vi "BitShifting.vi"(11 "register in":u16) -> (0 "4-1 Error":bool, 1 "8-5 Error":bool, 2 "12-9 Error":bool, 3 "16-13 Error":bool, 4 "SystemFault":bool, 5 "Warning":bool)   [LabVIEW 2014]
panel:
  out "16-13":u8
  out "12-9":u8
  out "8-5":u8
  out "1-4":u8
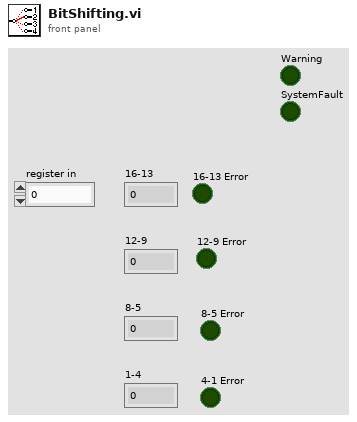
[diagram p1: front panel]
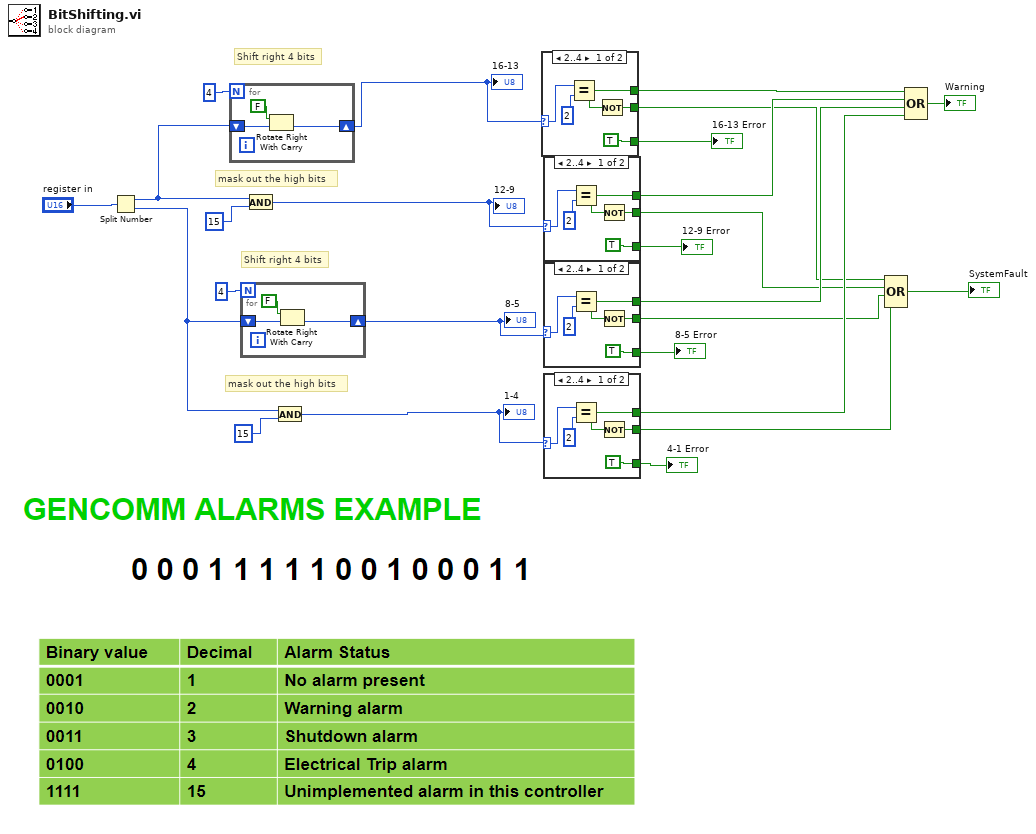
[diagram p0: block diagram]
diagram:
  # "mask out the high bits"
  # "Shift right 4 bits"
  # "mask out the high bits"
  # "Shift right 4 bits"
  n1 = Split Number(x="register in") -> (hi(x)=w21:u8, lo(x)=w25:u8)
  n2 = for {
    N: 4 -> [_]
    shift-right: [w27] -> w17
    shift-left: w21 -> [w28]
    n3 = Rotate Right With Carry(2:w28, 3:FALSE ("carry")) -> (0:w27:u8)  [unwired: 1 out]
  }
  "16-13" <- w17
  n4 = for {
    N: 4 -> [_]
    shift-right: [w30] -> w16
    shift-left: w25 -> [w31]
    n5 = Rotate Right With Carry(2:w31, 3:FALSE ("carry")) -> (0:w30:u8)  [unwired: 1 out]
  }
  "8-5" <- w16
  n6 = And(x=w21, y=u8 15) -> (x .and. y?=w1:u8)
  "12-9" <- w1
  n7 = And(x=w25, y=u8 15) -> (x .and. y?=w15:u8)
  "1-4" <- w15
  n8 = case shown="2..4" w17 {
    selector: w17 -> [w35 _]
    tunnel: [TRUE _] -> w18
    tunnel: [w33 _] -> w12
    tunnel: [w32 _] -> w8
    frame 2..4 {
      n9 = Equal?(x=w35, y=u8 2) -> (x = y?=w33:bool)
      n10 = Not(x=w33) -> (.not. x?=w32:bool)
    }
    frame Default {
    }
  }
  "16-13 Error" <- w18
  n11 = case shown="2..4" w1 {
    selector: w1 -> [w40 _]
    tunnel: [TRUE _] -> w3
    tunnel: [w38 _] -> w11
    tunnel: [w37 _] -> w7
    frame 2..4 {
      n12 = Equal?(x=w40, y=u8 2) -> (x = y?=w38:bool)
      n13 = Not(x=w38) -> (.not. x?=w37:bool)
    }
    frame Default {
    }
  }
  "12-9 Error" <- w3
  n14 = case shown="2..4" w16 {
    selector: w16 -> [w45 _]
    tunnel: [TRUE _] -> w2
    tunnel: [w43 _] -> w10
    tunnel: [w42 _] -> w6
    frame 2..4 {
      n15 = Equal?(x=w45, y=u8 2) -> (x = y?=w43:bool)
      n16 = Not(x=w43) -> (.not. x?=w42:bool)
    }
    frame Default {
    }
  }
  "8-5 Error" <- w2
  n17 = case shown="2..4" w15 {
    selector: w15 -> [w50 _]
    tunnel: [TRUE _] -> w14
    tunnel: [w48 _] -> w9
    tunnel: [w47 _] -> w5
    frame 2..4 {
      n18 = Equal?(x=w50, y=u8 2) -> (x = y?=w48:bool)
      n19 = Not(x=w48) -> (.not. x?=w47:bool)
    }
    frame Default {
    }
  }
  "4-1 Error" <- w14
  n20 = Compound Arithmetic op=OR(w8, w7, w6, w5) -> (→"SystemFault":bool)
  n21 = Compound Arithmetic op=OR(w12, w11, w10, w9) -> (→"Warning":bool)
